vi "Update-map-display.vi"(8 "error in":errorcluster, 10 "Map":T1, 11 "Mapping":refnum<vi>) -> (0 "error IO":errorcluster)   [LabVIEW 2013, in "CameraVision.lvlib" / "CV-Mapping.lvclass"]
uses:
  CV-Mapping.lvclass
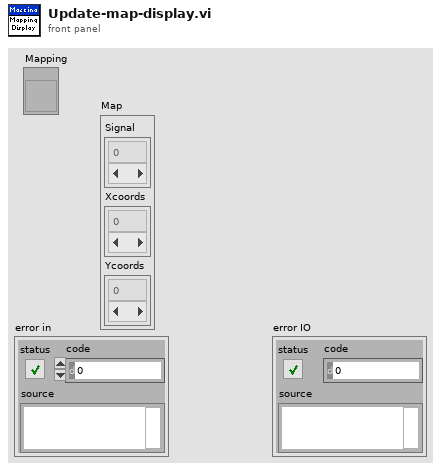
[diagram p1: front panel]
types:
  T1 = cluster{"Signal":sgl[], "Xcoords":sgl[], "Ycoords":sgl[]}
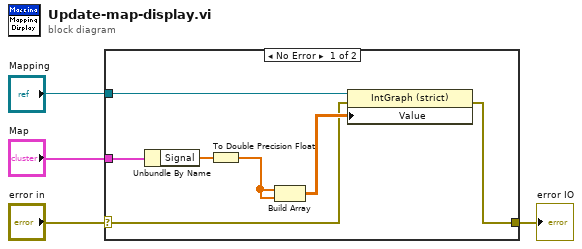
[diagram p0: block diagram]
diagram:
  n1 = case shown="No Error" "error in" {
    selector: "error in" -> [w6 w12]
    tunnel: [w11 w12] -> w4
    tunnel: "Mapping" -> [w9 _]
    tunnel: "Map" -> [w10 _]
    frame No Error {
      n2 = Unbundle By Name(w10) -> ("Signal"=w8:sgl[])
      n3 = To Double Precision Float(number=w8) -> (double precision float=w5:dbl[])
      n4 = Build Array(w5, w5) -> (w7:dbl[][])
      n5 = property class="IntGraph (strict)"(reference=w9, error in=w6, "Value"=w7) -> (error out=w11:errorcluster)  [unwired: 1 out]
    }
    frame Error {
    }
  }
  "error IO" <- w4
